vi "Get State.vi"(8 "error in (no error)":errorcluster, 11 "Spectrum Recorder in":refnum<class "Spectrum Recorder too.lvclass">) -> (0 "error out":errorcluster, 1 "Result ready":bool, 2 "Armed":bool, 3 "Spectrum Recorder out":refnum<class "Spectrum Recorder too.lvclass">)   [LabVIEW 2016]
uses:
  Spectrum Recorder too.lvclass
  C:/github/Measure_core/Instrument Actor/Instrument Actor.lvclass
  C:/github/Measure_core/Worker/Worker.lvclass
  C:/github/Measure_core/Template Module/Template Module.lvclass
  C:/Program Files/National Instruments/LabVIEW 2016/vi.lib/ActorFramework/Actor/Actor.lvclass
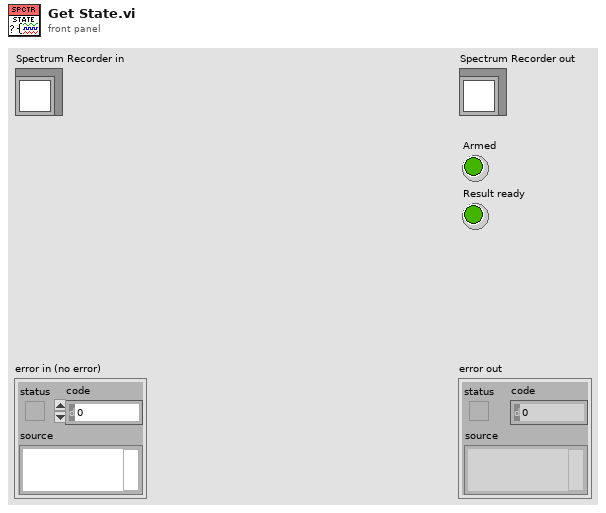
[diagram p1: front panel]
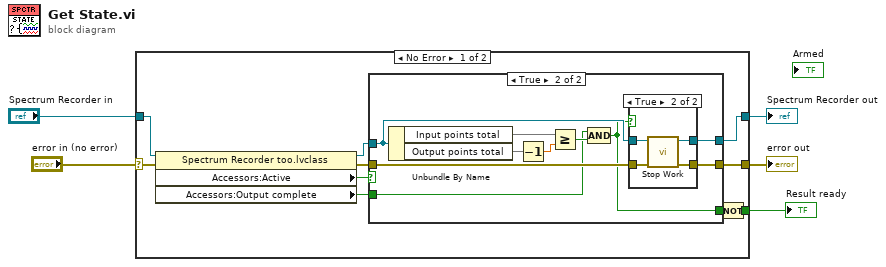
[diagram p0: block diagram]
diagram:
  n1 = case shown="No Error" "error in (no error)" {
    selector: "error in (no error)" -> [w14 w36]
    tunnel: [w13 w36] -> w4
    tunnel: [w15 w35] -> w2
    tunnel: "Spectrum Recorder in" -> [w11 w35]
    tunnel: [w6 _] -> w1
    frame No Error {
      n2 = property class="Spectrum Recorder too.lvclass"(reference=w11, error in=w14) -> (reference out=w10:refnum<class "Spectrum Recorder too.lvclass">, error out=w12:errorcluster, "Accessors:Active"=w9:bool, "Accessors:Output complete"=w8:bool)
      n3 = case shown="True" w9 {
        tunnel: w10 -> [w17 w25]
        tunnel: w12 -> [w18 w24]
        tunnel: [w18 w23] -> w13
        tunnel: [w17 w22] -> w15
        tunnel: w8 -> [w16 w20]
        tunnel: [w16 w19] -> w7
        frame False {
        }
        frame True {
          n4 = Unbundle By Name(w25) -> ("Input points total"=w28, "Output points total"=w27)
          n5 = Decrement(x=w27) -> (x-1=w21:dbl)
          n6 = Greater Or Equal?(x=w28, y=w21) -> (x >= y?=w26:bool)
          n7 = Compound Arithmetic op=AND(w20, w26) -> (w19:bool)
          n8 = case shown="True" w19 {
            tunnel: w25 -> [w30 w34]
            tunnel: w24 -> [w29 w33]
            tunnel: [w29 w32] -> w23
            tunnel: [w30 w31] -> w22
            frame False {
            }
            frame True {
              n9 = call-dynamic "Stop Work.vi"("error in (no error)"=w33, "Spectrum Recorder in"=w34) -> ("error out"=w32:errorcluster, "Spectrum Recorder out"=w31:refnum<class "Spectrum Recorder too.lvclass">)  [unwired: 8 in]
            }
          }
        }
      }
      n10 = Not(x=w7) -> (.not. x?=w6:bool)
    }
    frame Error {
    }
  }
  "error out" <- w4
  "Spectrum Recorder out" <- w2
  "Result ready" <- w1
